vi "Tab Control - Get Tab By Name.vi"(8 "error in (no error)":errorcluster, 10 "page caption (empty)":string, 11 "page control ref":refnum<vi>) -> (0 "error out":errorcluster, 2 "page caption out":string, 3 "page ref out":refnum<vi>)   [LabVIEW 2020]
doc: "Gets page reference for page given by name or returns selected page ref if no name provided."
uses:
  <vilib>/Utility/error.llb/Error Cluster From Error Code.vi
  <vilib>/ErrorRing/Error Ring.xnode
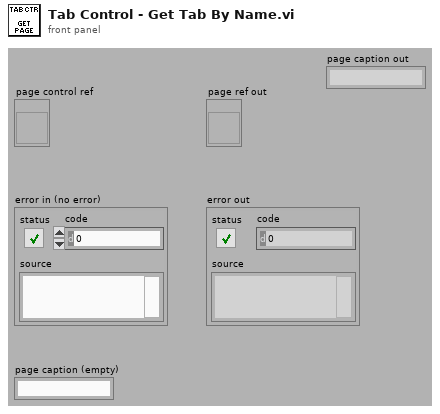
[diagram p1: front panel]
types:
  T1 = enum32{"abs", "abs fr", "fr/N", "fr*M/N", "fr*R", "fix"}
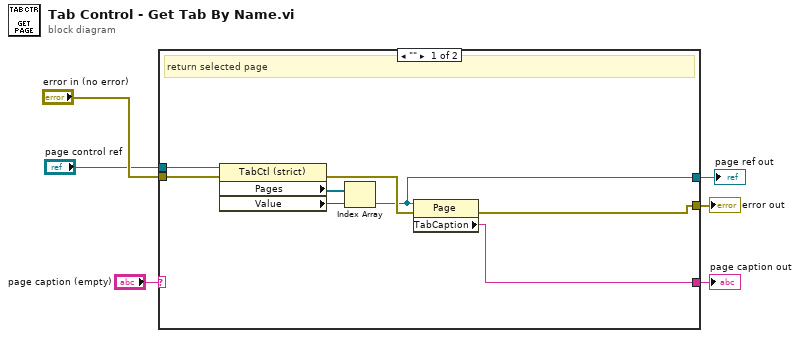
[diagram p0: block diagram]
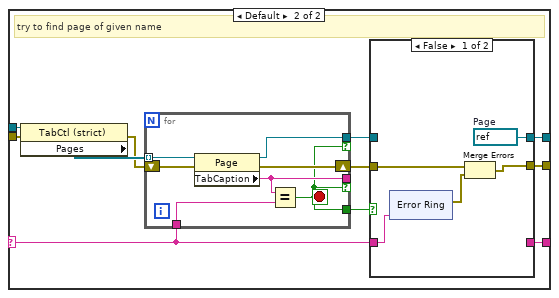
[diagram p2: hidden frame]
diagram:
  n1 = case shown="\"\"" "page caption (empty)" {
    selector: "page caption (empty)" -> [_ w16]
    tunnel: "page control ref" -> [w13 w25]
    tunnel: [w7 w19] -> w6
    tunnel: [w8 w18] -> w5
    tunnel: "error in (no error)" -> [w14 w17]
    tunnel: [w9 w15] -> w1
    frame "" {
      # "return selected page"
      n2 = property class="TabCtl (strict)"(reference=w13, error in=w14) -> (error out=w10:errorcluster, "Pages"=w11:refnum<vi>[], "Value"=w12:T1)  [unwired: 1 out]
      n3 = Index Array(array=w11, index=w12) -> (element=w7:refnum<vi>)
      n4 = property class="Page"(reference=w7, error in=w10) -> (error out=w8:errorcluster, "TabCaption"=w9:string)  [unwired: 1 out]
    }
    frame Default {
      # "try to find page of given name"
      n5 = property class="TabCtl (strict)"(reference=w25, error in=w17) -> (error out=w23:errorcluster, "Pages"=w24:refnum<vi>[])  [unwired: 1 out]
      n6 = for {
        tunnel: w24 -> [w47] mode=indexing
        tunnel: [w45] -> _ if=w41
        tunnel: [w41] -> w22
        shift-right: [w44] -> w21
        shift-left: w23 -> [w46]
        tunnel: w16 -> [w43]
        tunnel: [w42] -> w20 if=w41
        stop <- w41 stop-if-true
        n7 = property class="Page"(reference=w47, error in=w46) -> (reference out=w42:refnum<vi>, error out=w44:errorcluster, "TabCaption"=w45:string)
        n8 = Equal?(x=w45, y=w43) -> (x = y?=w41:bool)
      }
      n9 = case shown="False" w22 {
        tunnel: w21 -> [w30 w40]
        tunnel: [w28 w40] -> w18
        tunnel: [w26 w39] -> w19
        tunnel: w20 -> [_ w39]
        tunnel: w16 -> [w27 w38]
        tunnel: [_ w38] -> w15
        frame False {
          w26 = refnum<vi> refnum  # Page
          n10 = xnode "Error Ring"("parameter 0"=w27) -> ("error out"=w29:errorcluster)
          n11 = Merge Errors(w30, w29) -> (w28:errorcluster)
        }
        frame True {
        }
      }
    }
  }
  "page ref out" <- w6
  "error out" <- w5
  "page caption out" <- w1
